vi "find_element(variant).vi"(8 "error in (no error)":errorcluster, 10 "name":string, 11 "data store (in)":variant) -> (0 "error out":errorcluster, 1 "values":cluster{"name":string, "address":string}, 2 "found":bool, 3 "data store (out)":variant)   [LabVIEW 2016]
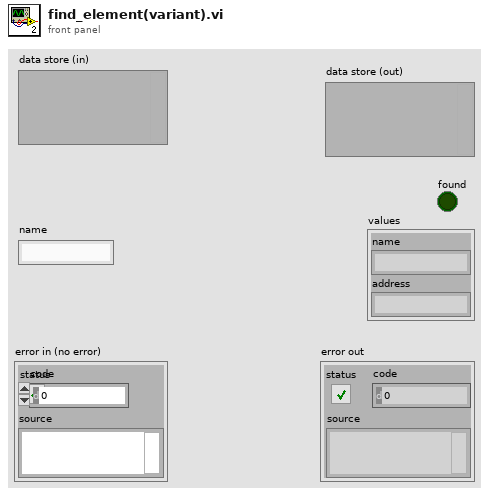
[diagram p1: front panel]
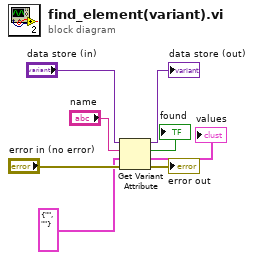
[diagram p0: block diagram]
diagram:
  n1 = Get Variant Attribute(Variant="data store (in)", name="name", default value (empty Variant)=cluster{"name":string, "address":string} {"name"="", "address"=""} ("element"), error in="error in (no error)") -> (duplicate Variant=→"data store (out)":variant, found=→"found":bool, value=→"values":cluster{"name":string, "address":string}, error out=→"error out":errorcluster)
